vi "TestGetNumber.vi"(7 "LabVIEW Web Service Request":refnum<class "Web Request.lvclass">) -> (0 "Group":cluster{"A":i32, "B":i32}, 1 "DataArray":i32[](array[numeric]), 2 "RND":i32, 3 "CNT":i32)   [LabVIEW 2015]
uses:
  <vilib>/wsapi/Web Request.lvclass
panel:
  # "Use the Web Service Request input terminal to call the VIs on the Web Services palette. Do not remove it from the connector pane unless you don't need access to the palette."
  # "Each additional control wired to the connector pane will be available as an input in the URL. To include an indicator in terminal-mode output (the default setting), it must also be wired to the connector pane."
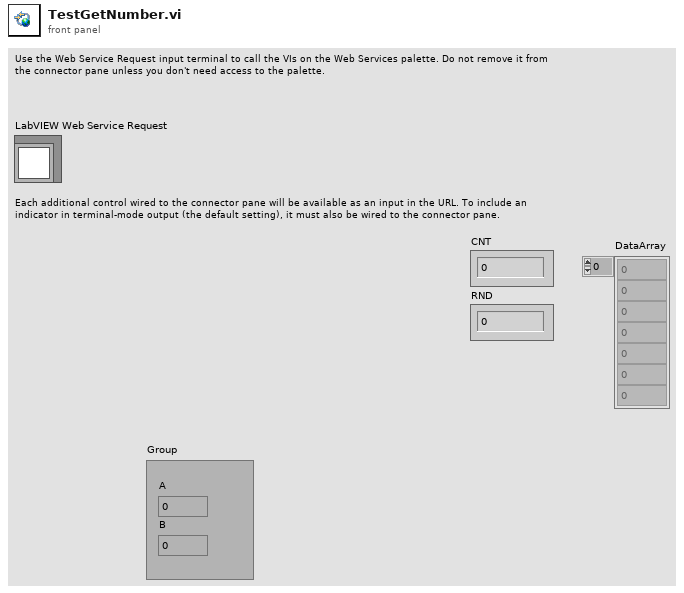
[diagram p1: front panel]
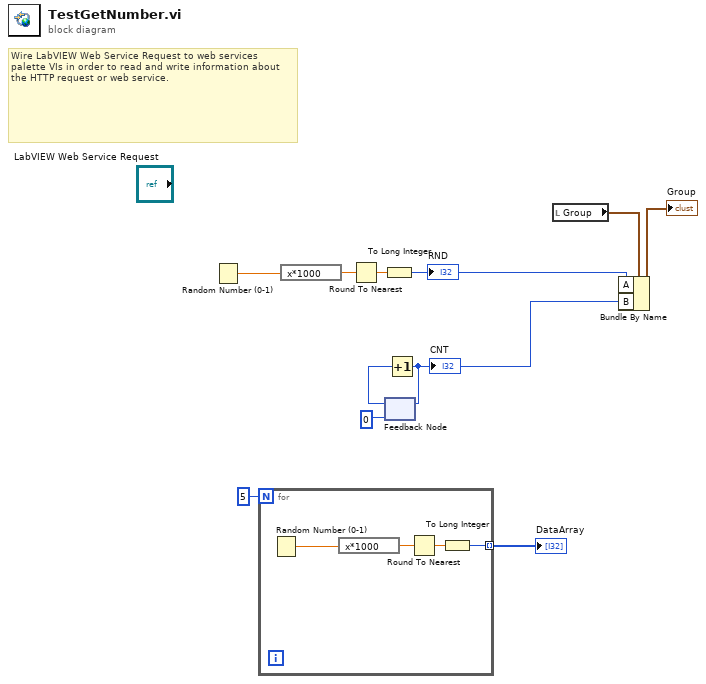
[diagram p0: block diagram]
diagram:
  # "Wire LabVIEW Web Service Request to web services palette VIs in order to read and write information about the HTTP request or web service."
  n1 = Random Number (0-1)() -> (number: 0 to 1=w10:dbl)
  n2 = for {
    N: 5 -> [_]
    tunnel: [w12] -> w7 mode=indexing
    n3 = Random Number (0-1)() -> (number: 0 to 1=w13:dbl)
    n4 = expression code="x*1000"(w13) -> (w14:dbl)
    n5 = Round To Nearest(number=w14) -> (nearest integer value=w15:dbl)
    n6 = To Long Integer(number=w15) -> (32bit integer=w12:i32)
  }
  "DataArray" <- w7
  n7 = expression code="x*1000"(w10) -> (w9:dbl)
  n8 = Round To Nearest(number=w9) -> (nearest integer value=w8:dbl)
  n9 = To Long Integer(number=w8) -> (32bit integer=w3:i32)
  "RND" <- w3
  n10 = feedback #1(0) -> (w11:i32)
  n11 = Increment(x=w11) -> (x+1=w2:i32)
  "CNT" <- w2
  n12 = feedback-in #1(w2) -> ()
  n13 = local read "Group"() -> (w5:cluster{"A":i32, "B":i32})
  n14 = Bundle By Name(cluster=w5, "A"=w3, "B"=w2) -> (→"Group":cluster{"A":i32, "B":i32})
